vi "SingleEncoderData.vi"(6 "Reset?":bool=TRUE, 8 "Tick Constant":dbl, 10 "Rate":dbl, 11 "Distance":dbl) -> (3 "Encoder Data":T1 {"Ticks" format="%#.6g"})   [LabVIEW 2014]
uses:
  Encoder Values.ctl
  <vilib>/addons/control/pid/pid.llb/PID Control Input Filter (DBL).vi
  <vilib>/addons/control/pid/NI_PID_pid.lvlib
panel:
  in  "Encoder Values TD":T1 {"Ticks" format="%#.6g"}
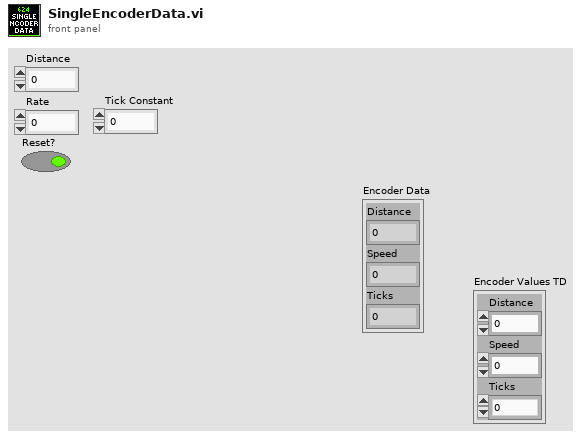
[diagram p1: front panel]
types:
  T1 = typedef "Encoder Values.ctl" = cluster{"Distance":dbl, "Speed":dbl, "Ticks":dbl}
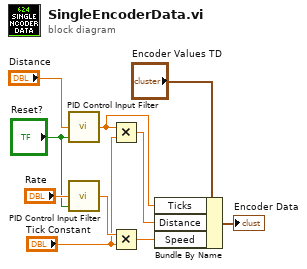
[diagram p0: block diagram]
diagram:
  n1 = call-poly <vilib>:"PID Control Input Filter.vi"("reinitialize? (F)"="Reset?", "input"="Distance") -> ("output"=w1:dbl)  [unwired: 3 in]
  n2 = call-poly <vilib>:"PID Control Input Filter.vi"("reinitialize? (F)"="Reset?", "input"="Rate") -> ("output"=w10:dbl)  [unwired: 3 in]
  n3 = Multiply(x=w1, y="Tick Constant") -> (x*y=w5:dbl)
  n4 = Multiply(x=w10, y="Tick Constant") -> (x*y=w4:dbl)
  n5 = Bundle By Name(cluster="Encoder Values TD", "Ticks"=w1, "Distance"=w5, "Speed"=w4) -> (→"Encoder Data":T1)
